vi "SECoP-registerUserError.vi"(8 "error in (no error)":errorcluster, 9 "message text":string, 10 "SECoP-Error":string, 11 "DLL path (in)":T2) -> (0 "error out":errorcluster, 2 "registered SECoP error":T1 items=["warn: missing properties"=4, "warn: buffer too small"=3, "warn: custom property"=2, "warn: no description"=1, "success"=0, "error: unknown command"=-1, "error: invalid name"=-2, "error: invalid node"=-3, "error: invalid module"=-4, "error: invalid parameter"=-5, "error: invalid property"=-6, "error: invalid command"=-7, "error: not implemented"=-8, "error: readonly"=-9, "error: no data"=-10, "error: no memory"=-11, "error: not initialized"=-12, "error: invalid value"=-13, "error: missing mandatory prop"=-14, "error: no setter/getter"=-15, "error: no setter"=-16, "error: no getter"=-17, "error: name already in use"=-18], 3 "DLL path (out)":T2)   [LabVIEW 2023, in "SECoP.lvlib"]
doc: "Call <b>\"SECoP-registerUserError.vi\"</b> to register your own SECoP errors with own text description. This function will return an unused \"SECoP-error.ctl\" code, which you should use with \"SECoP-putCommandAnswer.vi\", \"SECoP-putCommandAnswer_2.vi\".\n\n<b>DLL path</b> input and output of cluster from \"SECoP-Initialize.vi\"\n<b>SECoP-Error</b> SECoP error string (starting with letter or underscore and using letters, digits and underscore only)\n<b>message text</b> human readable description\n<b>registered SECoP error</b> new registered \"SECoP-error.ctl\" code"
uses:
  SECoP.lvlib
  SECoP-libraries.ctl
  SECoP-error.ctl
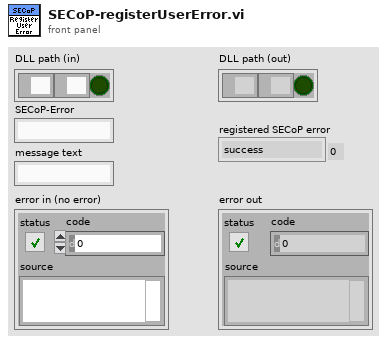
[diagram p1: front panel]
types:
  T1 = typedef "SECoP.lvlib/SECoP-error.ctl" = i32
  T2 = typedef "SECoP.lvlib/SECoP-libraries.ctl" = cluster{"serverDLL":path, "variantDLL":path, "cleanup_mode":bool}
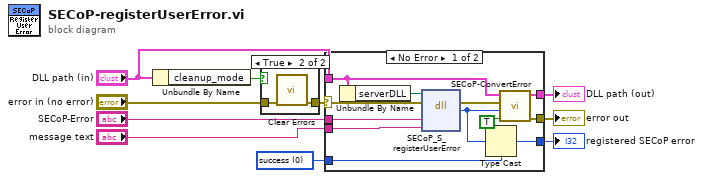
[diagram p0: block diagram]
diagram:
  w1 = T1 0 items=["warn: missing properties"=4, "warn: buffer too small"=3, "warn: custom property"=2, "warn: no description"=1, "success"=0, "error: unknown command"=-1, "error: invalid name"=-2, "error: invalid node"=-3, "error: invalid module"=-4, "error: invalid parameter"=-5, "error: invalid property"=-6, "error: invalid command"=-7, "error: not implemented"=-8, "error: readonly"=-9, "error: no data"=-10, "error: no memory"=-11, "error: not initialized"=-12, "error: invalid value"=-13, "error: missing mandatory prop"=-14, "error: no setter/getter"=-15, "error: no setter"=-16, "error: no getter"=-17, "error: name already in use"=-18] ("registered SECoP error")
  n1 = Unbundle By Name("DLL path (in)") -> ("cleanup_mode"=w7:bool)
  n2 = case shown="True" w7 {
    tunnel: "error in (no error)" -> [w11 w13]
    tunnel: [w11 w12] -> w6
    frame False {
    }
    frame True {
      n3 = call <vilib>:"Clear Errors.vi"("error in (no error)"=w13) -> ("error out"=w12:errorcluster)  [unwired: 5 in, 1 out]
    }
  }
  n4 = case shown="No Error" w6 {
    selector: w6 -> [w24 w27]
    tunnel: "DLL path (in)" -> [w21 w28]
    tunnel: [w20 w28] -> w9
    tunnel: [w18 w27] -> w10
    tunnel: "SECoP-Error" -> [w23 _]
    tunnel: "message text" -> [w22 _]
    tunnel: [w15 w26] -> w2
    tunnel: w1 -> [w14 w26]
    frame No Error {
      n5 = Unbundle By Name(w21) -> ("serverDLL"=w25:path)
      n6 = dll-call lib="?" fn="SECoP_S_registerUserError"(path in=w25, error in=w24, "szSECoPerror"=w23, "szMessageText"=w22) -> (error out=w19:errorcluster, "return type"=w16:i32)  [unwired: 3 in, 1 out]
      n7 = Type Cast(type=w14, x=w16) -> (*(type *) &x=w15:T1)
      n8 = call "SECoP-ConvertError.vi"("return is boolean"=TRUE, "return code"=w16, "error in (no error)"=w19, "DLL path (in)"=w21) -> ("error out"=w18:errorcluster, "DLL path (out)"=w20:T2)  [unwired: 6 in]
    }
    frame Error {
    }
  }
  "DLL path (out)" <- w9
  "error out" <- w10
  "registered SECoP error" <- w2
